vi "Stop Core.vi"(10 "final error code":i32, 11 "Cooler UI with Events in":refnum<class "Cooler UI with Events.lvclass">) -> (3 "Cooler UI with Events out":refnum<class "Cooler UI with Events.lvclass">)   [LabVIEW 2012, in "Cooler UI.lvlib" / "Cooler UI with Events.lvclass"]
doc: "(<B>Filename</B>: Actor Framework.lvlib:Actor.lvclass:Stop Core.vi)\n\nDefines what the actor does before it stops. Use the <B>final error code</B> input to determine whether the actor shut down in response to an error.\n\nBy default, this method does nothing. A descendant class may override it to define behavior, such as shutting down any processes the actor initiated in its override of the Actor Core method."
uses:
  Cooler UI with Events.lvclass
  <vilib>/ActorFramework/Actor/Actor.lvclass
  Cooler UI with Events.lvclass/Cooler UI with Events.ctl
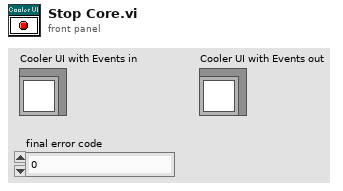
[diagram p1: front panel]
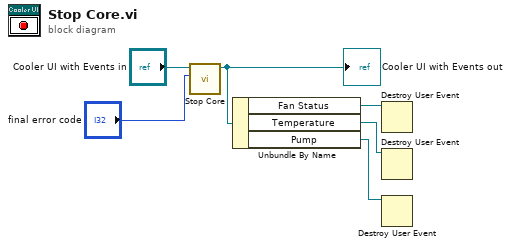
[diagram p0: block diagram]
diagram:
  n1 = call-parent "Stop Core.vi"("final error code"="final error code", "Actor in"="Cooler UI with Events in") -> ("Actor out"=w4:refnum<class "Cooler UI with Events.lvclass">)  [unwired: 9 in]
  "Cooler UI with Events out" <- w4
  n2 = Unbundle By Name(w4) -> ("Fan Status"=w3:refnum<user-event>, "Temperature"=w2:refnum<user-event>, "Pump"=w1:refnum<user-event>)
  n3 = Destroy User Event(user event=w3) -> ()  [unwired: 1 in, 1 out]
  n4 = Destroy User Event(user event=w2) -> ()  [unwired: 1 in, 1 out]
  n5 = Destroy User Event(user event=w1) -> ()  [unwired: 1 in, 1 out]
